vi "BRig_Host__Loop_Producer__UploadClosedLoop.vi"(11 "String":string) -> ()   [LabVIEW 2014]
uses:
  <vilib>/WebDAVClient/Advanced/Put File.vi
  <vilib>/WebDAVClient/Advanced/Get File.vi
  <vilib>/WebDAVClient/NI_WebDAV.lvlib
panel:
  out "text 2":string
  out "Get Copy":bool
  out "Sent":bool
  out "text":string
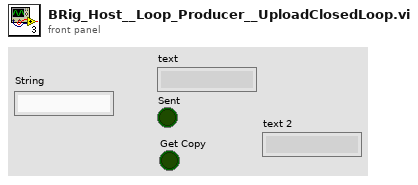
[diagram p1: front panel]
types:
  T1 = typedef "NI_WebDAV.lvlib/SessionHandle.ctl" = refnum<k1>
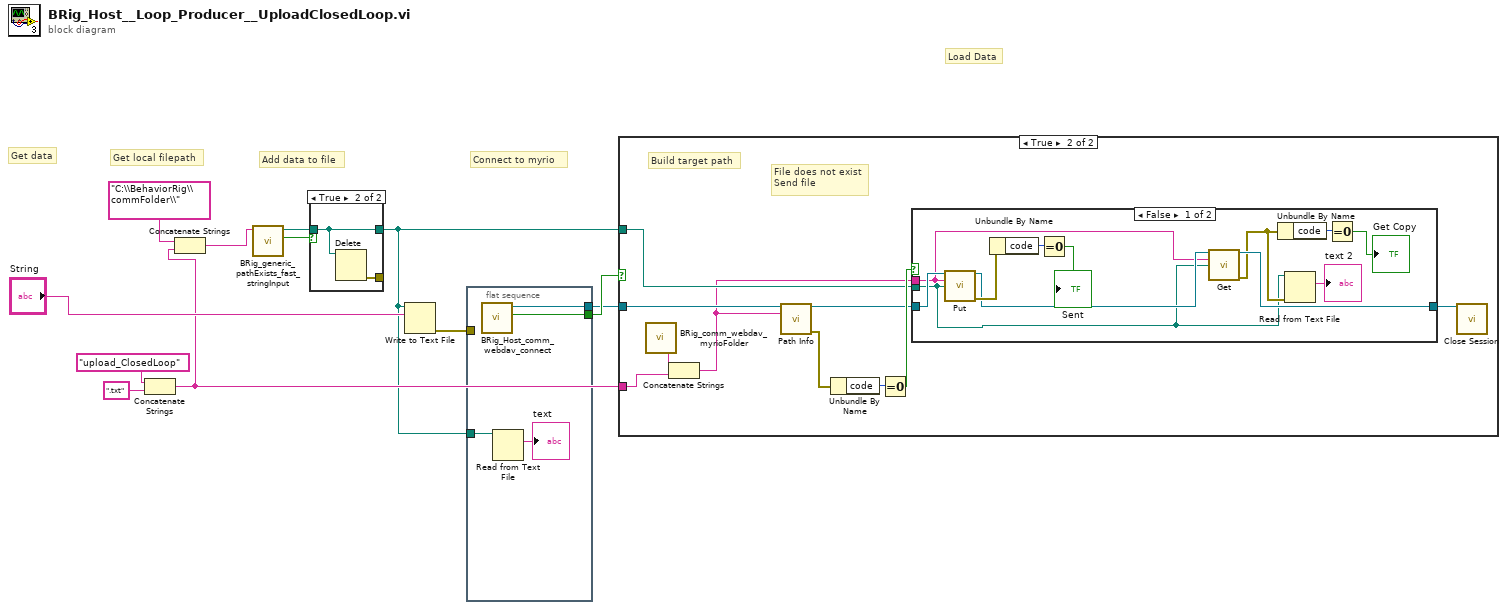
[diagram p0: block diagram]
diagram:
  # "Connect to myrio"
  # "Add data to file"
  # "Get local filepath"
  # "Get data"
  # "Load Data"
  n1 = Concatenate Strings("upload_ClosedLoop" ("string"), ".txt" ("string")) -> (w3:string)
  n2 = Concatenate Strings("C:\\BehaviorRig\\commFolder\\", w3) -> (w2:string)
  n3 = call "BRig_generic_pathExists_fast_stringInput.vi"("input_filePath"=w2) -> ("output_Iexist"=w12:bool, "output_filePath"=w11:path)  [unwired: 8 in, 1 out]
  n4 = case shown="True" w12 {
    tunnel: w11 -> [w13 w14]
    tunnel: [_ w15] -> _
    tunnel: [w13 w14] -> w1
    frame False {
    }
    frame True {
      n5 = Delete(path (use dialog)=w14) -> (error out=w15:errorcluster)  [unwired: 4 in, 2 out]
    }
  }
  n6 = Write to Text File(file (use dialog)=w1, text="String") -> (error out=w9:errorcluster)  [unwired: 2 in, 2 out]
  n7 = flat-sequence {
    tunnel: w9 -> [_]
    tunnel: [w19] -> w8
    tunnel: [w18] -> w7
    tunnel: w1 -> [w17]
    frame #0 {
      n8 = call "BRig_Host_comm_webdav_connect.vi"() -> ("output_Iconnected"=w19:bool, "output_hSession"=w18:T1)  [unwired: 9 in, 1 out]
      n9 = Read from Text File(file (use dialog)=w17) -> (text=→"text":string)  [unwired: 3 in, 3 out]
    }
  }
  n10 = case shown="True" w8 {
    tunnel: w7 -> [_ w27]
    tunnel: w1 -> [_ w21]
    tunnel: w3 -> [_ w28]
    frame False {
    }
    frame True {
      # "File does not exist\nSend file"
      # "Build target path"
      n11 = call "BRig_comm_webdav_myrioFolder.vi"() -> ("output_myrioFolder"=w29:string)  [unwired: 11 in]
      n12 = Concatenate Strings(w29, w28) -> (w20:string)
      n13 = call <vilib>:"Path Info.vi"("session handle"=w27, "relative uri"=w20) -> ("session handle out"=w23:T1, "error out"=w25:errorcluster)  [unwired: 10 in, 2 out]
      n14 = Unbundle By Name(w25) -> ("code"=w26:i32)
      n15 = Equal To 0?(x=w26) -> (x = 0?=w24:bool)
      n16 = case shown="False" w24 {
        tunnel: w23 -> [w41 w42]
        tunnel: [w36 w42] -> w22
        tunnel: w21 -> [w30 _]
        tunnel: w20 -> [w35 _]
        frame False {
          n17 = call-poly <vilib>:"Put.vi"("session handle"=w41, "relative uri"=w35, "local file path"=w30) -> ("session handle out"=w37:T1, "error out"=w39:errorcluster)  [unwired: 10 in, 1 out]
          n18 = Unbundle By Name(w39) -> ("code"=w40:i32)
          n19 = Equal To 0?(x=w40) -> (x = 0?=→"Sent":bool)
          n20 = call-poly <vilib>:"Get.vi"("session handle"=w37, "relative uri"=w35, "local file path"=w30) -> ("session handle out"=w36:T1, "error out"=w31:errorcluster)  [unwired: 10 in, 1 out]
          n21 = Unbundle By Name(w31) -> ("code"=w34:i32)
          n22 = Read from Text File(file (use dialog)=w30, error in=w31) -> (text=→"text 2":string)  [unwired: 2 in, 3 out]
          n23 = Equal To 0?(x=w34) -> (x = 0?=→"Get Copy":bool)
        }
        frame True {
        }
      }
      n24 = call <vilib>:"Close Session.vi"("session handle"=w22) -> ()  [unwired: 14 in, 1 out]
    }
  }
